vi "Replace minimum time.vi"(11 "Array":T1(array[cluster])) -> (3 "Array 2":T1(array[cluster]))   [LabVIEW 2012]
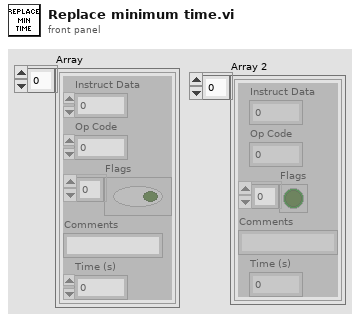
[diagram p1: front panel]
types:
  T1 = cluster{"Instruct Data":i32, "Op Code":i32, "Flags":bool[], "Comments":string, "Time (s)":dbl}[]
  T2 = cluster{"Instruct Data":i32, "Op Code":i32, "Flags":bool[], "Comments":string, "Time (s)":dbl}
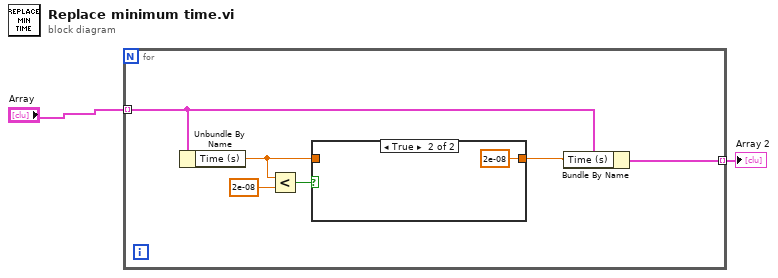
[diagram p0: block diagram]
diagram:
  n1 = for {
    tunnel: "Array" -> [w5] mode=indexing
    tunnel: [w3] -> w1 mode=indexing
    n2 = Unbundle By Name(w5) -> ("Time (s)"=w6:dbl)
    n3 = Less?(x=w6, y=2e-08) -> (x < y?=w8:bool)
    n4 = case shown="True" w8 {
      tunnel: w6 -> [w9 _]
      tunnel: [w9 2e-08 ("Time (s)")] -> w4
      frame False {
      }
      frame True {
      }
    }
    n5 = Bundle By Name(cluster=w5, "Time (s)"=w4) -> (w3:T2)
  }
  "Array 2" <- w1
